vi "Read Configuration.vi"(8 "error in (no error)":errorcluster, 11 "RandomNumberLogger Controller in":refnum<class "RandomNumberLogger Controller.lvclass">) -> (0 "error out":errorcluster, 2 "Configuration":T1, 3 "RandomNumberLogger Controller out":refnum<class "RandomNumberLogger Controller.lvclass">)   [LabVIEW 2020, in "RandomNumberLogger.lvlib" / "RandomNumberLogger Controller.lvclass"]
doc: "<b>Read Configuration</b>\nThis method directly returns the <b>Configuration.ct</b> stored in the class data of this plugin's controller."
uses:
  RandomNumberLogger Controller.lvclass
  RandomNumberLogger Controller.lvclass/RandomNumberLogger Controller.ctl
  PE/Configuration.ctl
  PE/RandomNumberLogger.lvclass
panel:
  # "#via_ignore"
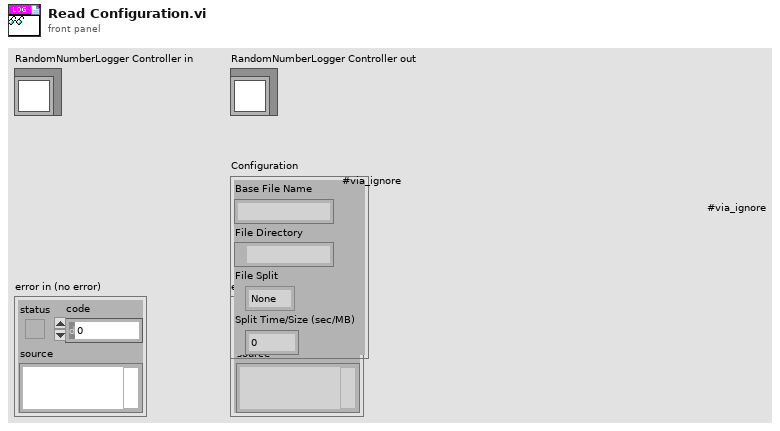
[diagram p1: front panel]
types:
  T1 = typedef "RandomNumberLogger.lvlib/RandomNumberLogger.lvclass/Configuration.ctl" = cluster{"Base File Name":string, "File Directory":path, "File Split":enum16{"None", "Time", "Size"}, "Split Time/Size (sec/MB)":dbl}
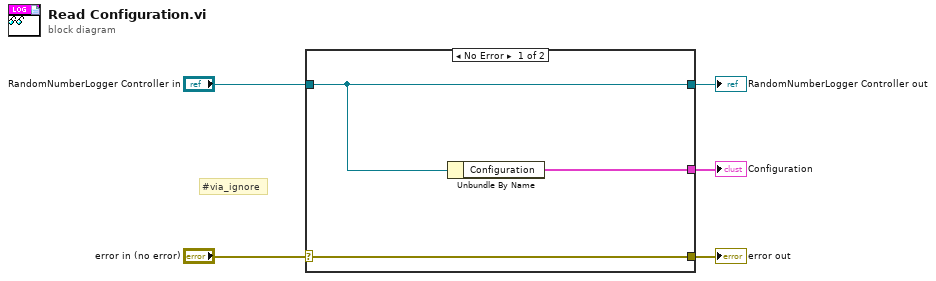
[diagram p0: block diagram]
diagram:
  # "#via_ignore"
  n1 = case shown="No Error" "error in (no error)" {
    selector: "error in (no error)" -> [w8 w9]
    tunnel: [w8 w9] -> w4
    tunnel: [w6 w10] -> w2
    tunnel: "RandomNumberLogger Controller in" -> [w6 w10]
    tunnel: [w7 _] -> w1
    frame No Error {
      n2 = Unbundle By Name(w6) -> ("Configuration"=w7:T1)
    }
    frame Error {
    }
  }
  "error out" <- w4
  "RandomNumberLogger Controller out" <- w2
  "Configuration" <- w1
